vi "B-Scan (Relative [FLR]).vi"(7 "Micropulse # In":i32, 9 "Scan definition":T1={"Scan Length"=0.0, "Inspection Resolution"=280.0, "Direction"=enum."Forwards"} {"Inspection Resolution" format="%#_6f"; "Scan Length" format="%#_6f"}, 10 "Axis No.":u8=1 min=1 max=4, 11 "scan data info":T3 {"Error Message" format="%04x"; "Message Header" format="%04x"; "IP"."MIP location" format="%#.0f"; "IP"."Location" format="%#.0f"; "PRF" format="%.0fHz"}) -> (0 "Update Display?":bool, 1 "B-Scan In Progress?":bool, 2 "B-Scan index":i32, 3 "B-Scan Out":u16[][](array[numeric]))   [LabVIEW 2026, in "MicroPulse_Driver.lvlib"]
uses:
  MicroPulse_Driver.lvlib
  Data/Datatypes/MP - scan data info.ctl
  Data/Datatypes/MP - data output format.ctl
  Data/Datatypes/MP - retain scan.ctl
  Data/Datatypes/MP - axis positions (LLC).ctl
  Data/Datatypes/MP - fly scan range (relative).ctl
  Data/Datatypes/MP - inspection direction (relative).ctl
  Low Level/FGV - B-Scan Active - Action [Enum].ctl
  <instrlib>/Micropulse/Micropulse.lvlib
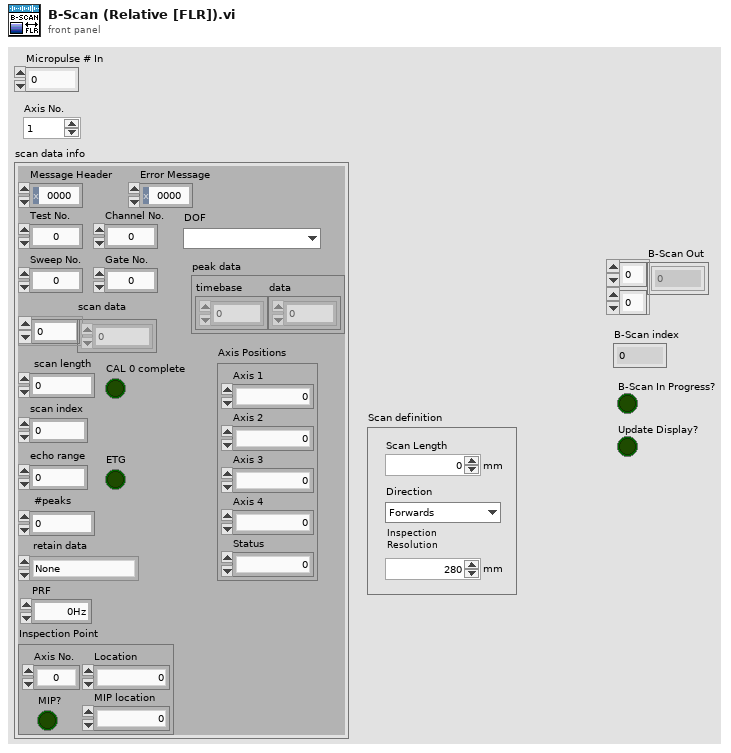
[diagram p1: front panel]
types:
  T1 = typedef "Micropulse.lvlib/MP - fly scan range (relative).ctl" = cluster{"Scan Length":dbl, "Inspection Resolution":dbl, "Direction":T2}
  T2 = typedef "Micropulse.lvlib/MP - inspection direction (relative).ctl" = enum16{"Forwards", "Backwards", "Bidirectional"}
  T3 = typedef "Micropulse.lvlib/MP - scan data info.ctl" = cluster{"Message Header":u16, "Error Message":u16, "Test No.":u32, "Channel No.":u8, "Sweep No.":u32, "Gate No.":u32, "DOF":T4, "retain data":T5, "scan data":u16[], "scan length":i32, "scan index":i32, "peak data":cluster{"timebase":u16[], "data":u16[]}, "#peaks":i32, "PRF":dbl, "IP":cluster{"Axis No.":u8, "Location":u32, "MIP location":u32, "MIP?":bool}, "echo range":u16, "ETG":bool, "CAL 0 complete":bool, "Axis Positions":T6}
  T4 = typedef "Micropulse.lvlib/MP - data output format.ctl" = enum16{"", "8-bit Mode", "10-bit Mode", "12-bit Mode", "16-bit Mode", "8-bit Log Mode", "12-bit Packed Mode"}
  T5 = typedef "Micropulse.lvlib/MP - retain scan.ctl" = enum16{"None", "Ascan", "Peaks"}
  T6 = typedef "Micropulse.lvlib/MP - axis positions (LLC).ctl" = cluster{"Axis 1":u32, "Axis 2":u32, "Axis 3":u32, "Axis 4":u32, "Status":u8}
  T7 = typedef "MicroPulse_Driver.lvlib/FGV - B-Scan Active - Action [Enum].ctl" = enum16{"Read", "Read & Reset Start Flag", "Start B-Scan", "B-Scan Finished"}
  T8 = cluster{"Lowest location":i32, "Highest location":i32}
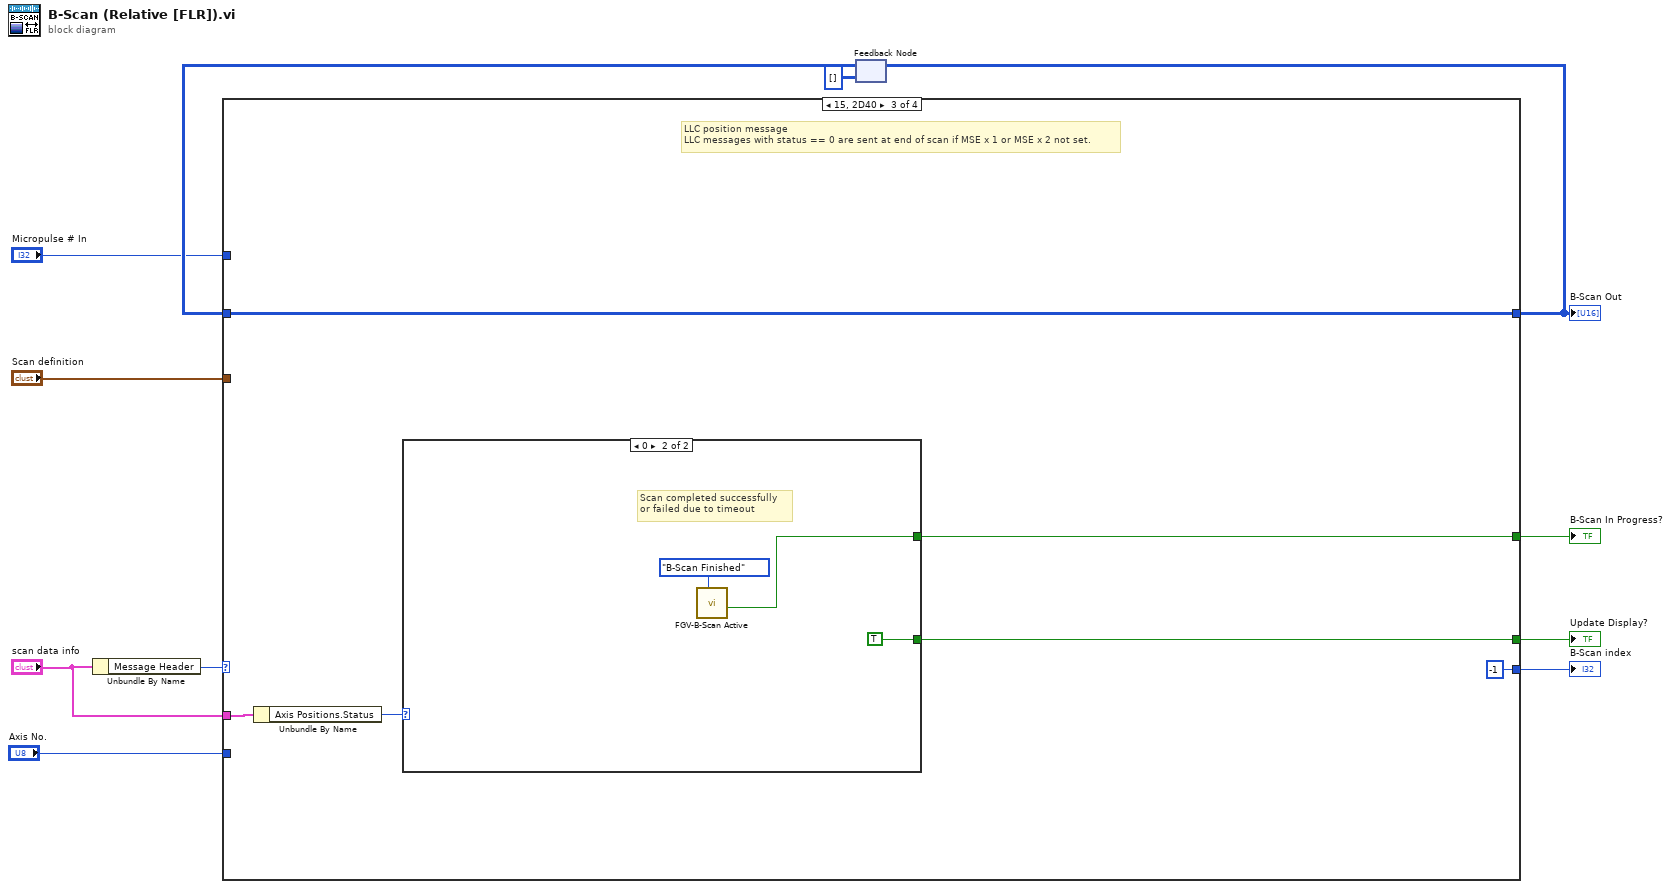
[diagram p0: block diagram]
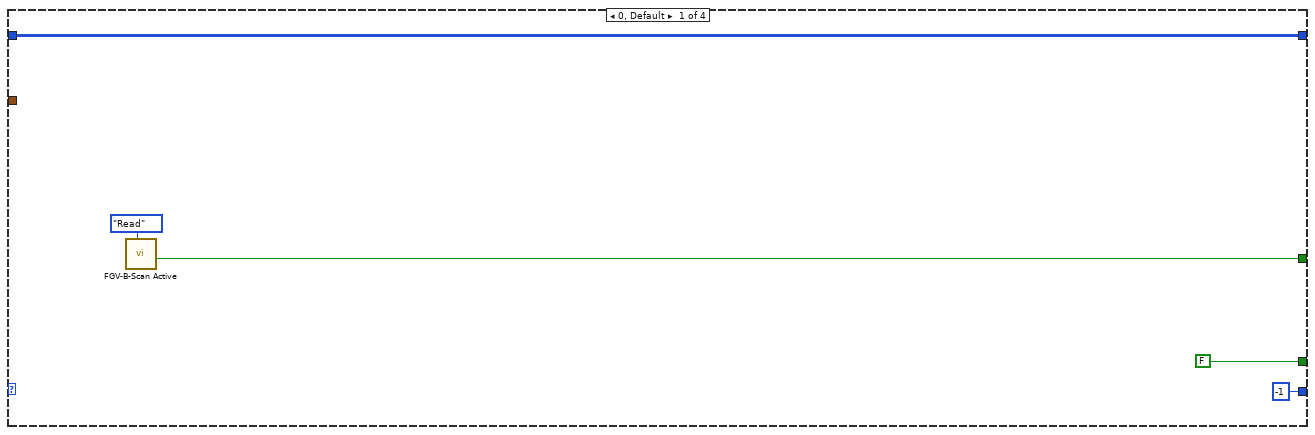
[diagram p2: hidden frame]
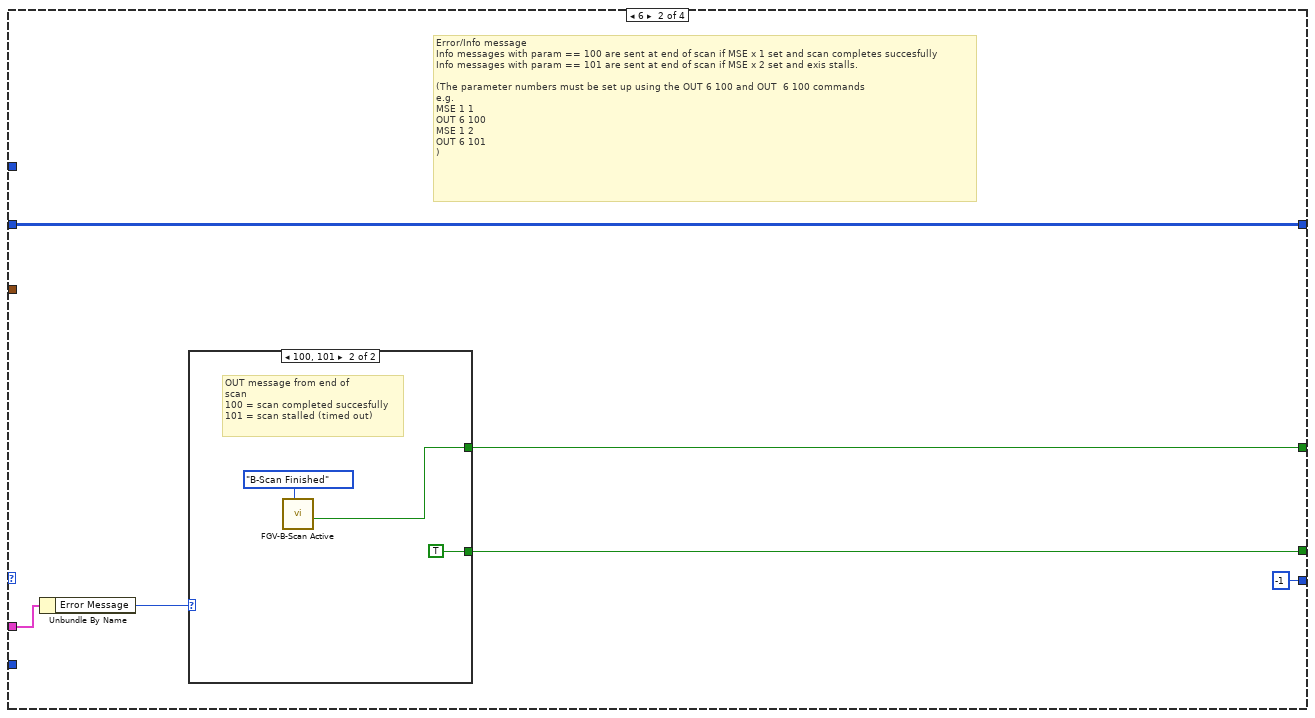
[diagram p3: hidden frame]
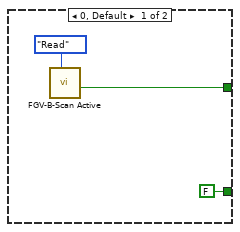
[diagram p4: hidden frame]
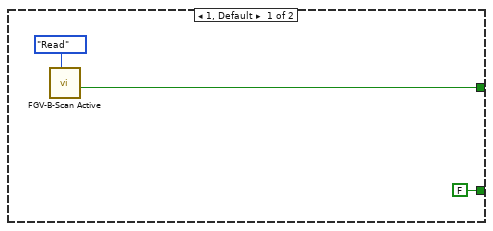
[diagram p5: hidden frame]
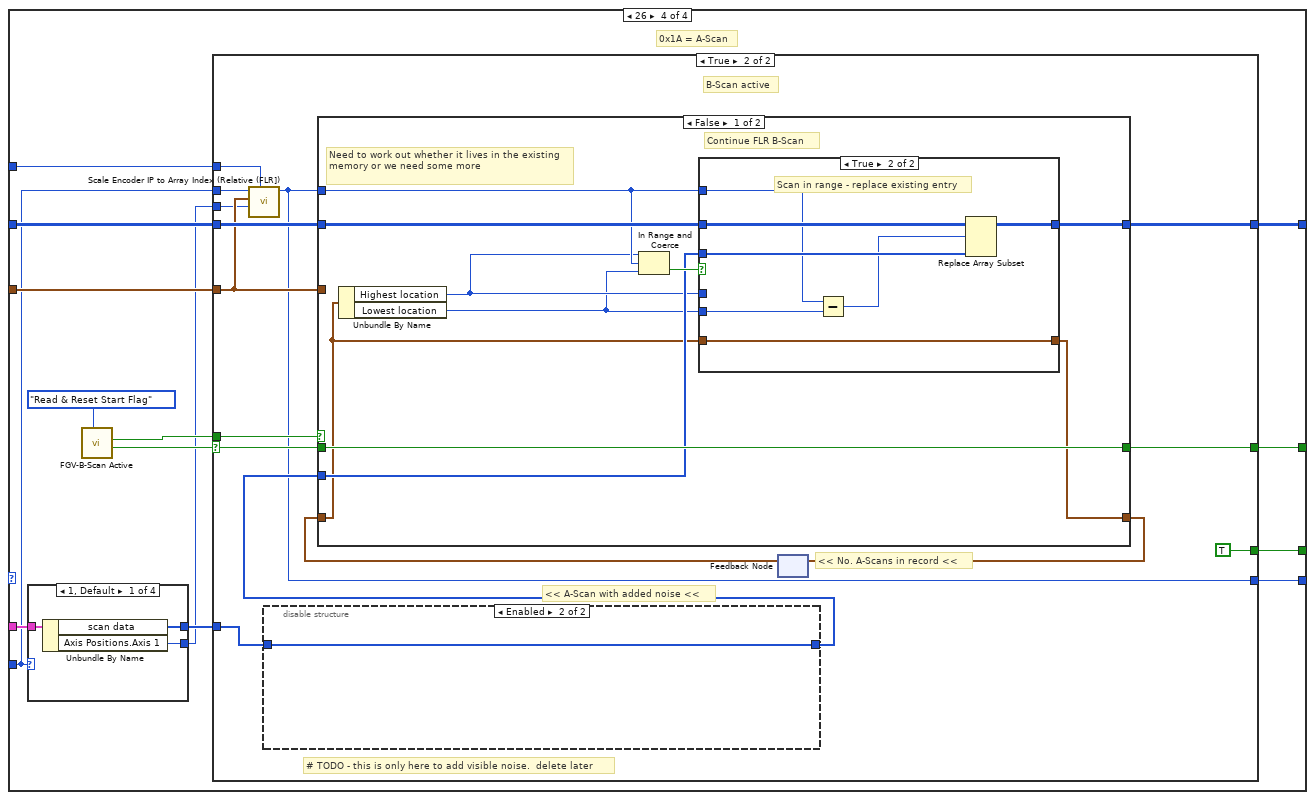
[diagram p6: hidden frame]
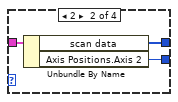
[diagram p7: hidden frame]
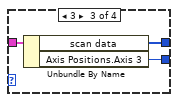
[diagram p8: hidden frame]
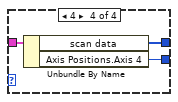
[diagram p9: hidden frame]
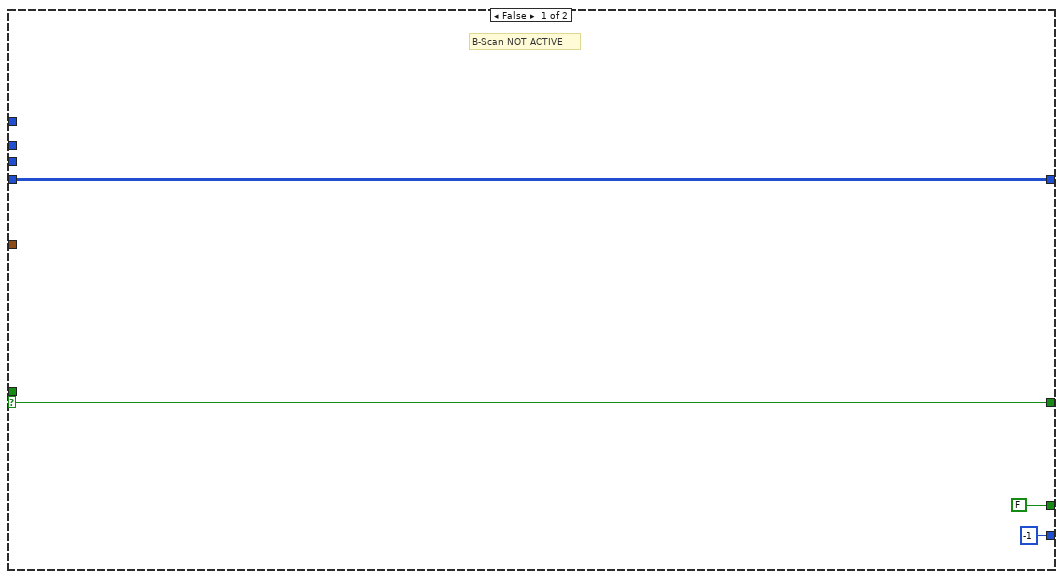
[diagram p10: hidden frame]
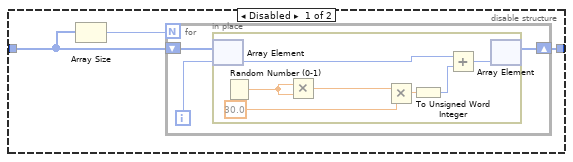
[diagram p11: hidden frame]
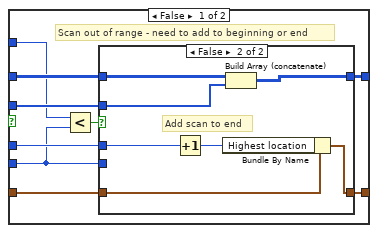
[diagram p12: hidden frame]
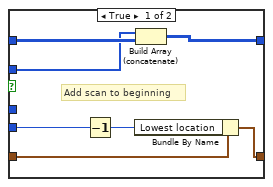
[diagram p13: hidden frame]
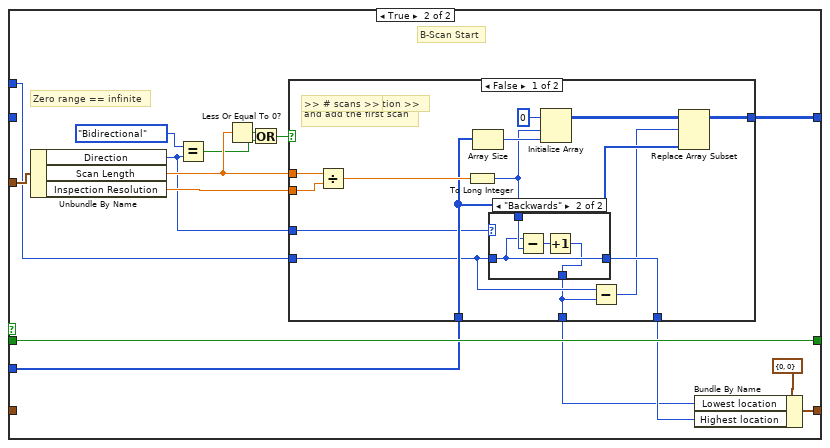
[diagram p14: hidden frame]
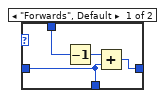
[diagram p15: hidden frame]
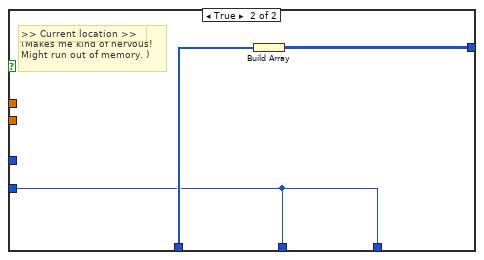
[diagram p16: hidden frame]
diagram:
  n1 = Unbundle By Name("scan data info") -> ("Message Header"=w11:u16)
  n2 = feedback #1(u16[][] []) -> (w7:u16[][])
  n3 = case shown="15, 2D40" w11 {
    tunnel: "scan data info" -> [_ w21 w33 w54]
    tunnel: "Scan definition" -> [_ _ _ w48]
    tunnel: [w16 w22 w34 w52] -> w8
    tunnel: w7 -> [w16 w22 w34 w51]
    tunnel: "Micropulse # In" -> [_ _ _ w47]
    tunnel: [w13 w19 w31 w50] -> w4
    tunnel: [FALSE w17 w29 w49] -> w3
    tunnel: "Axis No." -> [_ _ _ w42]
    tunnel: [-1 ("B-Scan index") -1 ("B-Scan index") -1 ("B-Scan index") w41] -> w1
    frame 0, Default {
      n4 = call "FGV-B-Scan Active.vi"("Action"=FGV_-_B-Scan_Active_-_Action_[Enum]."Read") -> ("B-Scan In Progress?"=w13:bool)  [unwired: 8 in, 2 out]
    }
    frame 6 {
      # "Error/Info message\nInfo messages with param == 100 are sent at end of scan if MSE x 1 set and scan completes succesfully\nInfo messages with param == 101 are sent at end of scan if MSE x 2 set and exis stalls.\n\n(The parameter numbers must be set up using the OUT 6 100 and OUT  6 100 commands \ne.g.\nMSE 1 1\nOUT 6 100\nMSE 1 2\nOUT 6 101\n)"
      n5 = Unbundle By Name(w21) -> ("Error Message"=w20:u16)
      n6 = case shown="100, 101" w20 {
        tunnel: [w24 w27] -> w19
        tunnel: [FALSE TRUE] -> w17
        frame 0, Default {
          n7 = call "FGV-B-Scan Active.vi"("Action"=FGV_-_B-Scan_Active_-_Action_[Enum]."Read") -> ("B-Scan In Progress?"=w24:bool)  [unwired: 8 in, 2 out]
        }
        frame 100, 101 {
          # "OUT message from end of\nscan\n100 = scan completed succesfully\n101 = scan stalled (timed out)"
          n8 = call "FGV-B-Scan Active.vi"("Action"=FGV_-_B-Scan_Active_-_Action_[Enum]."B-Scan Finished") -> ("B-Scan In Progress?"=w27:bool)  [unwired: 8 in, 2 out]
        }
      }
    }
    frame 21, 11584 {
      # "LLC position message\nLLC messages with status == 0 are sent at end of scan if MSE x 1 or MSE x 2 not set."
      n9 = Unbundle By Name(w33) -> ("Axis Positions.Status"=w32:u8)
      n10 = case shown="0" w32 {
        tunnel: [w36 w40] -> w31
        tunnel: [FALSE TRUE] -> w29
        frame 1, Default {
          n11 = call "FGV-B-Scan Active.vi"("Action"=FGV_-_B-Scan_Active_-_Action_[Enum]."Read") -> ("B-Scan In Progress?"=w36:bool)  [unwired: 8 in, 2 out]
        }
        frame 0 {
          # "Scan completed successfully\nor failed due to timeout"
          n12 = call "FGV-B-Scan Active.vi"("Action"=FGV_-_B-Scan_Active_-_Action_[Enum]."B-Scan Finished") -> ("B-Scan In Progress?"=w40:bool)  [unwired: 8 in, 2 out]
        }
      }
    }
    frame 26 {
      # "0x1A = A-Scan"
      n13 = case shown="1, Default" w42 {
        tunnel: w54 -> [w57 w60 w63 w66]
        tunnel: [w56 w59 w62 w65] -> w53
        tunnel: [w55 w58 w61 w64] -> w43
        frame 1, Default {
          n14 = Unbundle By Name(w57) -> ("scan data"=w56:u16[], "Axis Positions.Axis 1"=w55:u32)
        }
        frame 2 {
          n15 = Unbundle By Name(w60) -> ("scan data"=w59:u16[], "Axis Positions.Axis 2"=w58:u32)
        }
        frame 3 {
          n16 = Unbundle By Name(w63) -> ("scan data"=w62:u16[], "Axis Positions.Axis 3"=w61:u32)
        }
        frame 4 {
          n17 = Unbundle By Name(w66) -> ("scan data"=w65:u16[], "Axis Positions.Axis 4"=w64:u32)
        }
      }
      n18 = call "FGV-B-Scan Active.vi"("Action"=FGV_-_B-Scan_Active_-_Action_[Enum]."Read & Reset Start Flag") -> ("B-Scan In Progress?"=w44:bool, "B-Scan Start?"=w45:bool)  [unwired: 8 in, 1 out]
      n19 = case shown="True" w44 {
        selector: w44 -> [w69 w81]
        tunnel: w45 -> [_ w84]
        tunnel: w51 -> [w70 w85]
        tunnel: [w70 w78] -> w52
        tunnel: w53 -> [_ w77]
        tunnel: w48 -> [_ w74]
        tunnel: [w69 w82] -> w50
        tunnel: [FALSE TRUE] -> w49
        tunnel: w47 -> [_ w79]
        tunnel: w43 -> [_ w73]
        tunnel: w42 -> [_ w72]
        tunnel: [-1 ("B-Scan index") w71] -> w41
        frame False {
          # "B-Scan NOT ACTIVE"
        }
        frame True {
          # "<< A-Scan with added noise <<"
          # "B-Scan active"
          # "<< No. A-Scans in record <<"
          # "# TODO - this is only here to add visible noise.  delete later"
          n20 = call "Scale Encoder IP to Array Index (Relative (FLR]).vi"("Micropulse # In"=w79, "Inspection Point Location"=w73, "Scan definition"=w74, "Axis No."=w72) -> ("B-Scan index"=w71:i32)  [unwired: 7 in]
          n21 = disable-structure shown="Enabled" {
            disable-tunnel: w77 -> [w86 w99]
            disable-tunnel: [w87 w99] -> w76
            frame Disabled {
              n22 = Array Size(array=w86) -> (size(s)=w88:i32)
              n23 = for {
                N: w88 -> [_]
                shift-right: [w89] -> w87
                shift-left: w86 -> [w91]
                i -> [w90]
                n24 = in-place {
                  n25 = in-place-array #2(w91, w90) -> (w95:u16)
                  n26 = Random Number (0-1)() -> (number: 0 to 1=w92:dbl)
                  n27 = Multiply(x=w92, y=w92) -> (x*y=w93:dbl)
                  n28 = Multiply(x=w93, y=30.0) -> (x*y=w97:dbl)
                  n29 = To Unsigned Word Integer(number=w97) -> (unsigned 16bit integer=w96:u16)
                  n30 = Add(x=w95, y=w96) -> (x+y=w94:u16)
                  n31 = in-place-array #2(w94) -> (w89:u16[])  [unwired: 1 out]
                }
              }
            }
            frame Enabled {
            }
          }
          n32 = feedback #3() -> (w83:T8)  [unwired: 1 in]
          n33 = case shown="False" w84 {
            tunnel: w85 -> [w109 _]
            tunnel: [w107 w155] -> w78
            tunnel: w74 -> [_ w154]
            tunnel: w71 -> [w105 w141]
            tunnel: w83 -> [w101 _]
            tunnel: [w108 w152] -> w82
            tunnel: w81 -> [w108 w152]
            tunnel: w76 -> [w104 w149]
            tunnel: [w100 w147] -> w75
            frame False {
              # "Continue FLR B-Scan"
              # "Need to work out whether it lives in the existing memory or we need some more"
              n34 = Unbundle By Name(w101) -> ("Highest location"=w103:i32, "Lowest location"=w102:i32)
              n35 = In Range and Coerce(upper limit=w103, x=w105, lower limit=w102) -> (In Range?=w106:bool)  [unwired: 1 out]
              n36 = case shown="True" w106 {
                tunnel: w109 -> [w118 w139]
                tunnel: [w117 w138] -> w107
                tunnel: w105 -> [w115 w136]
                tunnel: w104 -> [w116 w137]
                tunnel: w103 -> [w113 _]
                tunnel: w102 -> [w110 w133]
                tunnel: w101 -> [w112 w134]
                tunnel: [w111 w134] -> w100
                frame False {
                  # "Scan out of range - need to add to beginning or end"
                  n37 = Less?(x=w115, y=w110) -> (x < y?=w114:bool)
                  n38 = case shown="False" w114 {
                    tunnel: w118 -> [w120 w132]
                    tunnel: [w125 w131] -> w117
                    tunnel: w116 -> [w119 w130]
                    tunnel: w113 -> [_ w126]
                    tunnel: w110 -> [w123 _]
                    tunnel: w112 -> [w124 w129]
                    tunnel: [w121 w127] -> w111
                    frame True {
                      # "Add scan to beginning"
                      n39 = Decrement(x=w123) -> (x-1=w122:i32)
                      n40 = Bundle By Name(cluster=w124, "Lowest location"=w122) -> (w121:T8)
                      n41 = Build Array (concatenate)(w119, w120) -> (w125:u16[][])
                    }
                    frame False {
                      # "Add scan to end"
                      n42 = Increment(x=w126) -> (x+1=w128:i32)
                      n43 = Bundle By Name(cluster=w129, "Highest location"=w128) -> (w127:T8)
                      n44 = Build Array (concatenate)(w132, w130) -> (w131:u16[][])
                    }
                  }
                }
                frame True {
                  # "Scan in range - replace existing entry"
                  n45 = Subtract(x=w136, y=w133) -> (x-y=w135:i32)
                  n46 = Replace Array Subset(array=w139, new element=w137, index (row)=w135) -> (w138:u16[][])  [unwired: 1 in]
                }
              }
            }
            frame True {
              # "Zero range == infinite"
              # "B-Scan Start"
              n47 = Unbundle By Name(w154) -> ("Direction"=w143:T2, "Scan Length"=w151:dbl, "Inspection Resolution"=w153:dbl)
              n48 = Equal?(x=MP_-_inspection_direction_(relative)."Bidirectional", y=w143) -> (x = y?=w144:bool)
              n49 = Less Or Equal To 0?(x=w151) -> (x <= 0?=w150:bool)
              n50 = Or(x=w150, y=w144) -> (x .or. y?=w145:bool)
              n51 = case shown="False" w145 {
                tunnel: [w163 w180] -> w155
                tunnel: w153 -> [w168 _]
                tunnel: w151 -> [w166 _]
                tunnel: w149 -> [w162 w179]
                tunnel: w141 -> [w159 w178]
                tunnel: w143 -> [w160 _]
                tunnel: [w158 w178] -> w142
                tunnel: [w157 w178] -> w140
                frame False {
                  # ">> Current location >>"
                  # "Pre-allocate memory\nand add the first scan"
                  # ">> # scans >>"
                  n52 = Divide(x=w166, y=w168) -> (x/y=w167:dbl)
                  n53 = To Long Integer(number=w167) -> (32bit integer=w161:i32)
                  n54 = Array Size(array=w162) -> (size(s)=w165:i32)
                  n55 = case shown="\"Backwards\"" w160 {
                    tunnel: w159 -> [w170 w175]
                    tunnel: w161 -> [w172 w177]
                    tunnel: [w171 w175] -> w158
                    tunnel: [w170 w174] -> w157
                    frame "Forwards", Default {
                      n56 = Decrement(x=w172) -> (x-1=w173:i32)
                      n57 = Add(x=w173, y=w170) -> (x+y=w171:i32)
                    }
                    frame "Backwards" {
                      n58 = Subtract(x=w175, y=w177) -> (x-y=w176:i32)
                      n59 = Increment(x=w176) -> (x+1=w174:i32)
                    }
                  }
                  n60 = Initialize Array(u16 0 ("index"), w161, w165) -> (w164:u16[][])
                  n61 = Subtract(x=w159, y=w157) -> (x-y=w156:i32)
                  n62 = Replace Array Subset(array=w164, new element=w162, index (row)=w156) -> (w163:u16[][])  [unwired: 1 in]
                }
                frame True {
                  # ">> Current location >>"
                  # "Infinite range.\n(Makes me kind of nervous!\nMight run out of memory. )"
                  n63 = Build Array(w179) -> (w180:u16[][])
                }
              }
              n64 = Bundle By Name(cluster=T8 {"Lowest location"=0, "Highest location"=0} ("input cluster"), "Lowest location"=w140, "Highest location"=w142) -> (w147:T8)
            }
          }
          n65 = feedback-in #3(w75) -> ()
        }
      }
    }
  }
  "B-Scan Out" <- w8
  "Update Display?" <- w3
  "B-Scan In Progress?" <- w4
  "B-Scan index" <- w1
  n66 = feedback-in #1(w8) -> ()
